vi "sub_solve1DArray.vi"(9 "type":enum16{"row", "column"}(ring), 10 "solver (in)":T1[][](array[typedef]), 11 "puzzle":string[][](array[string])) -> (2 "solver (out)":T1[][](array[typedef]), 3 "puzzle (out)":string[][](array[string]))   [LabVIEW 2018]
uses:
  cell.ctl
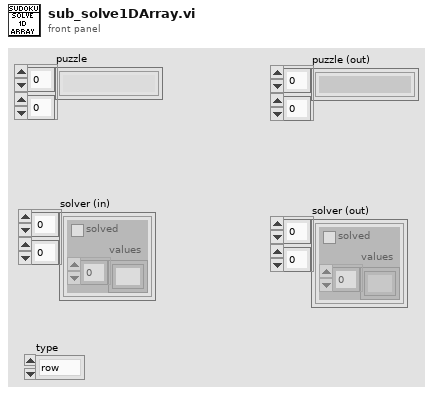
[diagram p1: front panel]
types:
  T1 = typedef "cell.ctl" = cluster{"solved":bool, "values":string[]}
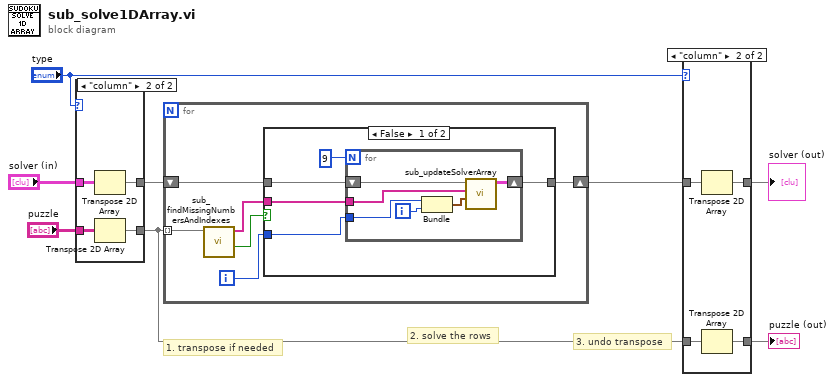
[diagram p0: block diagram]
diagram:
  # "3. undo transpose"
  # "2. solve the rows"
  # "1. transpose if needed"
  n1 = case shown="\"column\"" "type" {
    tunnel: "puzzle" -> [w10 w14]
    tunnel: [w10 w13] -> w4
    tunnel: "solver (in)" -> [w9 w12]
    tunnel: [w9 w11] -> w6
    frame "row", Default {
    }
    frame "column" {
      n2 = Transpose 2D Array(2D array=w12) -> (transposed array=w11:T1[][])
      n3 = Transpose 2D Array(2D array=w14) -> (transposed array=w13:string[][])
    }
  }
  n4 = for {
    tunnel: w4 -> [w20] mode=indexing
    shift-right: [w15] -> w5
    shift-left: w6 -> [w17]
    i -> [w16]
    n5 = call "sub_findMissingNumbersAndIndexes.vi"("row (in)"=w20) -> ("row solved"=w19:bool, "missing numbers"=w18:string[])  [unwired: 9 in]
    n6 = case shown="False" w19 {
      tunnel: w18 -> [w25 _]
      tunnel: w17 -> [w24 w32]
      tunnel: w16 -> [w22 _]
      tunnel: [w21 w32] -> w15
      frame False {
        n7 = for {
          N: 9 -> [_]
          tunnel: w25 -> [w27]
          tunnel: w22 -> [w30]
          shift-right: [w26] -> w21
          shift-left: w24 -> [w28]
          i -> [w31]
          n8 = Bundle(w30, w31) -> (w29:cluster{i32, i32})  [unwired: 1 in]
          n9 = call "sub_updateSolverArray.vi"("array index"=w29, "possible candidates"=w27, "solver (in)"=w28) -> ("solver (out)"=w26:cluster{"solved":bool, "values":string[]}[][])  [unwired: 8 in]
        }
      }
      frame True {
      }
    }
  }
  n10 = case shown="\"column\"" "type" {
    tunnel: w4 -> [w34 w38]
    tunnel: [w34 w37] -> w1
    tunnel: w5 -> [w33 w36]
    tunnel: [w33 w35] -> w2
    frame "row", Default {
    }
    frame "column" {
      n11 = Transpose 2D Array(2D array=w36) -> (transposed array=w35:T1[][])
      n12 = Transpose 2D Array(2D array=w38) -> (transposed array=w37:string[][])
    }
  }
  "solver (out)" <- w2
  "puzzle (out)" <- w1
